vi "Autonomous Independent.vi"() -> ()   [LabVIEW 2012]
doc: "This VI is called when autonomous begins, and will automatically be terminated when autonomous ends. You can carry out timed or sensor driven robot movement independently without needing to return to the caller."
uses:
  <vilib>/Rock Robotics/WPI/SafetyOutput/WPI_SafetyOutputConfigMenu.ctl
  <vilib>/Rock Robotics/WPI/Relay/WPI_RelayValue.ctl
  Extras/Global Data.vi
  <vilib>/Rock Robotics/WPI/RobotDrive/WPI_RobotDriveGetSetRefNum.vi
panel:
  out "1M in Distance":dbl
  out "Left Encdoer":string
  out "Right Encdoer":string
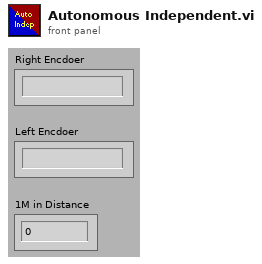
[diagram p1: front panel]
types:
  T1 = typedef "WPI_SafetyOutputConfigMenu.ctl" = enum16{"Enable", "Disable"}
  T2 = typedef "WPI_RelayDevRef.ctl" = cluster{"DevStatus":errorcluster, "Relay Channel":T3, "Digital Module":T4, "Relay Direction":T5}
  T3 = typedef "FPGA_DIORelayChannel.ctl" = enum8{"Relay 1", "Relay 2", "Relay 3", "Relay 4", "Relay 5", "Relay 6", "Relay 7", "Relay 8", "Invalid"}
  T4 = typedef "FPGA_TypedefDigitalModule.ctl" = enum16{"Digital Module 1", "Digital Module 2"}
  T5 = typedef "WPI_RelayDirection.ctl" = enum16{"Both directions", "Forward only", "Reverse only"}
  T6 = typedef "WPI_RobotDriveDevRef.ctl" = cluster{"DevStatus":errorcluster, "Motors[]":T7[], "Square Inputs":bool, "Max Output":dbl, "Isochronous":bool}
  T7 = typedef "WPI_MotorControlDeviceRef.ctl" = cluster{"DeviceStatus":errorcluster, "Type":enum16{"PWM", "CAN"}, "PWM":cluster{"Digital Module":T4, "PWM Channel":T8, "DeadBand":T9}, "CAN":cluster{"Device Number":u8, "Control Mode":T10, "Semaphore":T11, "Max Vout":dbl}, "Invert":bool, "TransformRef":T12, "InvTransformRef":T12}
  T8 = typedef "FPGA_DIOPWMChannel.ctl" = enum8{"PWM 1", "PWM 2", "PWM 3", "PWM 4", "PWM 5", "PWM 6", "PWM 7", "PWM 8", "PWM 9", "PWM 10", "Invalid"}
  T9 = typedef "WPI_PWMDeadband.ctl" = cluster{"Name":string, "maxPositivePwm":i32, "minPositivePwm":i32, "centerPwm":i32, "maxNegativePwm":i32, "minNegativePwm":i32, "angularRange":u16}
  T10 = typedef "WPI_CANJaguar_ControlMode.ctl" = enum8{"Percent VBus", "Current", "Speed", "Position", "Voltage"}
  T11 = typedef "Semaphore RefNum" = refnum<k1>
  T12 = typedef "WPI_PWMTransform_ConPane.ctl" = refnum<vi>
  T13 = typedef "WPI_DigitalInputDevRef.ctl" = cluster{"DevStatus":errorcluster, "DIO Channel":T14, "Digital Module":T4}
  T14 = typedef "FPGA_DIOChannel.ctl" = enum8{"DIO 1", "DIO 2", "DIO 3", "DIO 4", "DIO 5", "DIO 6", "DIO 7", "DIO 8", "DIO 9", "DIO 10", "DIO 11", "DIO 12", "DIO 13", "DIO 14", "Invalid"}
  T15 = typedef "WPI_RelayValue.ctl" = enum16{"Off", "On", "Forward", "Reverse"}
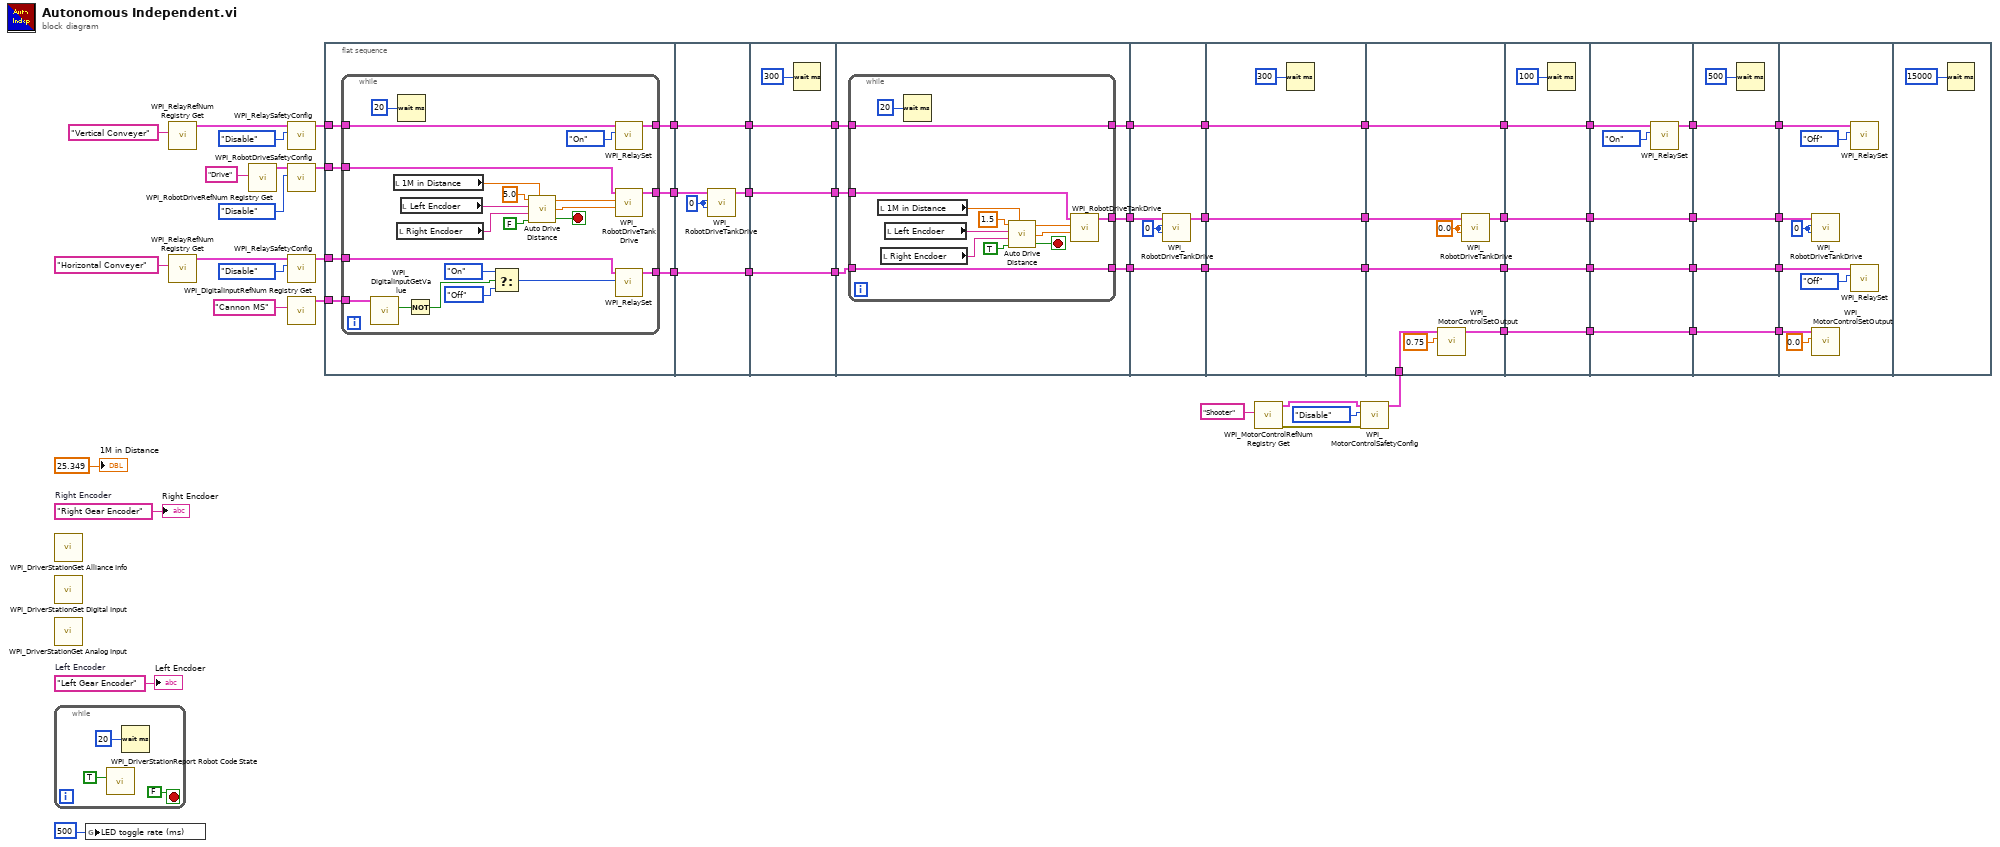
[diagram p0: block diagram]
diagram:
  w44 = "Left Gear Encoder"  # Left Encoder
  w45 = "Right Gear Encoder"  # Right Encoder
  n1 = call <vilib>:"WPI_DriverStationGet Alliance Info.vi"() -> ()  [unwired: 12 out]
  n2 = call <vilib>:"WPI_DriverStationGet Digital Input.vi"() -> ()  [unwired: 12 out]
  n3 = call <vilib>:"WPI_DriverStationGet Analog Input.vi"() -> ()  [unwired: 12 out]
  n4 = while {
    stop <- FALSE stop-if-true
    n5 = call <vilib>:"WPI_DriverStationReport Robot Code State.vi"("Autonomous"=TRUE) -> ()  [unwired: 10 in, 1 out]
    n6 = Wait (ms)(milliseconds to wait=u32 20) -> ()  [unwired: 1 out]
  }
  n7 = global write "Global Data.vi" "LED toggle rate (ms)"(u32 500 ("LED ms toggle rate")) -> ()
  n8 = call <vilib>:"WPI_RelayRefNum Registry Get.vi"("refnum name"="Vertical Conveyer") -> ("RelayDevRef"=w39:T2)  [unwired: 9 in, 1 out]
  n9 = call <vilib>:"WPI_RelayRefNum Registry Get.vi"("refnum name"="Horizontal Conveyer") -> ("RelayDevRef"=w42:T2)  [unwired: 9 in, 1 out]
  n10 = call <vilib>:"WPI_RobotDriveRefNum Registry Get.vi"("refnum name"="Drive") -> ("RobotDriveDevRef"=w54:T6)  [unwired: 9 in, 1 out]
  n11 = call <vilib>:"WPI_RelaySafetyConfig.vi"("mode"=WPI_SafetyOutputConfigMenu."Disable", "RelayDevRef"=w39) -> ("RelayDevRef"=w38:T2)  [unwired: 8 in, 1 out]
  n12 = call <vilib>:"WPI_RobotDriveSafetyConfig.vi"("mode"=WPI_SafetyOutputConfigMenu."Disable", "RobotDriveDevRef"=w54) -> ("RobotDriveDevRef"=w53:T6)  [unwired: 8 in, 1 out]
  n13 = call <vilib>:"WPI_RelaySafetyConfig.vi"("mode"=WPI_SafetyOutputConfigMenu."Disable", "RelayDevRef"=w42) -> ("RelayDevRef"=w37:T2)  [unwired: 8 in, 1 out]
  n14 = call <vilib>:"WPI_DigitalInputRefNum Registry Get.vi"("refnum name"="Cannon MS") -> ("DigitalInputDevRef"=w36:T13)  [unwired: 9 in, 1 out]
  n15 = flat-sequence {
    tunnel: w53 -> [w67]
    tunnel: w38 -> [w66]
    tunnel: w37 -> [w65]
    tunnel: w36 -> [w64]
    tunnel: [w63] -> w31
    tunnel: [w62] -> w30
    tunnel: [w61] -> w29
    tunnel: w31 -> [w93]
    tunnel: [w92] -> w51
    tunnel: w30 -> [w91]
    tunnel: w29 -> [w90]
    tunnel: [w91] -> w27
    tunnel: [w90] -> w25
    tunnel: w51 -> [w98]
    tunnel: [w98] -> w50
    tunnel: [w96] -> w28
    tunnel: w27 -> [w96]
    tunnel: [w95] -> w26
    tunnel: w25 -> [w95]
    tunnel: w50 -> [w103]
    tunnel: w28 -> [w104]
    tunnel: w26 -> [w102]
    tunnel: [w101] -> w24
    tunnel: [w100] -> w23
    tunnel: [w99] -> w22
    tunnel: [w122] -> w52
    tunnel: w24 -> [w118]
    tunnel: w23 -> [w119]
    tunnel: w22 -> [w120]
    tunnel: [w119] -> w21
    tunnel: [w118] -> w20
    tunnel: w52 -> [w123]
    tunnel: [w125] -> w3
    tunnel: w21 -> [w125]
    tunnel: [w124] -> w2
    tunnel: w20 -> [w124]
    tunnel: [w123] -> w1
    tunnel: [w134] -> w49
    tunnel: w16 -> [w132]
    tunnel: [w130] -> w15
    tunnel: [w129] -> w13
    tunnel: w3 -> [w129]
    tunnel: [w128] -> w11
    tunnel: w2 -> [w128]
    tunnel: w1 -> [w127]
    tunnel: w49 -> [w138]
    tunnel: [w138] -> w47
    tunnel: w15 -> [w135]
    tunnel: [w137] -> w14
    tunnel: w13 -> [w137]
    tunnel: [w136] -> w12
    tunnel: w11 -> [w136]
    tunnel: [w135] -> w4
    tunnel: w47 -> [w145]
    tunnel: [w145] -> w46
    tunnel: w14 -> [w143]
    tunnel: w12 -> [w141]
    tunnel: [w142] -> w9
    tunnel: [w141] -> w7
    tunnel: [w140] -> w5
    tunnel: w4 -> [w140]
    tunnel: w46 -> [w150]
    tunnel: [w150] -> w48
    tunnel: [w148] -> w10
    tunnel: w9 -> [w148]
    tunnel: [w147] -> w8
    tunnel: w7 -> [w147]
    tunnel: [w146] -> w6
    tunnel: w5 -> [w146]
    tunnel: w48 -> [w157]
    tunnel: w10 -> [w155]
    tunnel: w8 -> [w154]
    tunnel: w6 -> [w151]
    frame #0 {
      n16 = while {
        tunnel: [w89] -> w63
        tunnel: w67 -> [w84]
        tunnel: w66 -> [w79]
        tunnel: w65 -> [w78]
        tunnel: w64 -> [w76]
        tunnel: [w70] -> w62
        tunnel: [w69] -> w61
        stop <- w83 stop-if-true
        n17 = call <vilib>:"WPI_DigitalInputGetValue.vi"("DigitalInputDevRef"=w76) -> ("Value"=w75:bool)  [unwired: 8 in, 2 out]
        n18 = local read "1M in Distance"() -> (w81:dbl)
        n19 = local read "Right Encdoer"() -> (w87:string)
        n20 = Wait (ms)(milliseconds to wait=u32 20) -> ()  [unwired: 1 out]
        n21 = local read "Left Encdoer"() -> (w88:string)
        n22 = Not(x=w75) -> (.not. x?=w74:bool)
        n23 = Select(t=WPI_RelayValue."On" ("RelayValue"), s=w74, f=WPI_RelayValue."Off" ("RelayValue")) -> (s? t:f=w71:T15)
        n24 = call "Auto Drive Distance.vi"("Wanted Distance"=5.0 ("Numeric Control"), "Left Gear Encoder"=w88, "Right Gear Encoder"=w87, "Reverse?"=FALSE, "1M in Distance"=w81) -> ("Left Stick Value"=w86:dbl, "Right Stick Value"=w85:dbl, "Completed?"=w83:bool)
        n25 = call <vilib>:"WPI_RelaySet.vi"("RelayValue"=WPI_RelayValue."On", "RelayDevRef"=w79) -> ("RelayDevRef"=w70:T2)  [unwired: 8 in, 1 out]
        n26 = call <vilib>:"WPI_RobotDriveTankDrive.vi"("Right axis value"=w85, "Left axis value"=w86, "RobotDriveDevRef"=w84) -> ("RobotDriveDevRef"=w89:T6)  [unwired: 6 in, 2 out]
        n27 = call <vilib>:"WPI_RelaySet.vi"("RelayValue"=w71, "RelayDevRef"=w78) -> ("RelayDevRef"=w69:T2)  [unwired: 8 in, 1 out]
      }
    }
    frame #1 {
      w94 = 0
      n28 = call <vilib>:"WPI_RobotDriveTankDrive.vi"("Right axis value"=w94, "Left axis value"=w94, "RobotDriveDevRef"=w93) -> ("RobotDriveDevRef"=w92:T6)  [unwired: 6 in, 2 out]
    }
    frame #2 {
      n29 = Wait (ms)(milliseconds to wait=u32 300) -> ()  [unwired: 1 out]
    }
    frame #3 {
      n30 = while {
        tunnel: [w117] -> w99
        tunnel: w103 -> [w112]
        tunnel: w104 -> [w105]
        tunnel: w102 -> [w106]
        tunnel: [w106] -> w101
        tunnel: [w105] -> w100
        stop <- w111 stop-if-true
        n31 = local read "1M in Distance"() -> (w109:dbl)
        n32 = local read "Right Encdoer"() -> (w115:string)
        n33 = local read "Left Encdoer"() -> (w116:string)
        n34 = Wait (ms)(milliseconds to wait=u32 20) -> ()  [unwired: 1 out]
        n35 = call "Auto Drive Distance.vi"("Wanted Distance"=1.5 ("Numeric Control"), "Left Gear Encoder"=w116, "Right Gear Encoder"=w115, "Reverse?"=TRUE, "1M in Distance"=w109) -> ("Left Stick Value"=w114:dbl, "Right Stick Value"=w113:dbl, "Completed?"=w111:bool)
        n36 = call <vilib>:"WPI_RobotDriveTankDrive.vi"("Right axis value"=w113, "Left axis value"=w114, "RobotDriveDevRef"=w112) -> ("RobotDriveDevRef"=w117:T6)  [unwired: 6 in, 2 out]
      }
    }
    frame #4 {
      w121 = 0
      n37 = call <vilib>:"WPI_RobotDriveTankDrive.vi"("Right axis value"=w121, "Left axis value"=w121, "RobotDriveDevRef"=w120) -> ("RobotDriveDevRef"=w122:T6)  [unwired: 6 in, 2 out]
    }
    frame #5 {
      n38 = Wait (ms)(milliseconds to wait=u32 300) -> ()  [unwired: 1 out]
    }
    frame #6 {
      w133 = 0.0 ("Right axis value")
      n39 = call <vilib>:"WPI_MotorControlSetOutput.vi"("Output"=0.75, "MotorControlDevRef"=w132) -> ("MotorControlDevRef"=w130:T7)  [unwired: 7 in, 2 out]
      n40 = call <vilib>:"WPI_RobotDriveTankDrive.vi"("Right axis value"=w133, "Left axis value"=w133, "RobotDriveDevRef"=w127) -> ("RobotDriveDevRef"=w134:T6)  [unwired: 6 in, 2 out]
    }
    frame #7 {
      n41 = Wait (ms)(milliseconds to wait=u32 100) -> ()  [unwired: 1 out]
    }
    frame #8 {
      n42 = call <vilib>:"WPI_RelaySet.vi"("RelayValue"=WPI_RelayValue."On", "RelayDevRef"=w143) -> ("RelayDevRef"=w142:T2)  [unwired: 8 in, 1 out]
    }
    frame #9 {
      n43 = Wait (ms)(milliseconds to wait=u32 500) -> ()  [unwired: 1 out]
    }
    frame #10 {
      w158 = 0
      n44 = call <vilib>:"WPI_RobotDriveTankDrive.vi"("Right axis value"=w158, "Left axis value"=w158, "RobotDriveDevRef"=w157) -> ()  [unwired: 6 in, 3 out]
      n45 = call <vilib>:"WPI_MotorControlSetOutput.vi"("Output"=0.0, "MotorControlDevRef"=w151) -> ()  [unwired: 7 in, 3 out]
      n46 = call <vilib>:"WPI_RelaySet.vi"("RelayValue"=WPI_RelayValue."Off", "RelayDevRef"=w155) -> ()  [unwired: 8 in, 2 out]
      n47 = call <vilib>:"WPI_RelaySet.vi"("RelayValue"=WPI_RelayValue."Off", "RelayDevRef"=w154) -> ()  [unwired: 8 in, 2 out]
    }
    frame #11 {
      n48 = Wait (ms)(milliseconds to wait=u32 15000) -> ()  [unwired: 1 out]
    }
  }
  n49 = call <vilib>:"WPI_MotorControlRefNum Registry Get.vi"("refnum name"="Shooter") -> ("error out"=w18:errorcluster, "MotorControlDevRef"=w19:T7)  [unwired: 9 in]
  n50 = call <vilib>:"WPI_MotorControlSafetyConfig.vi"("error in (no error)"=w18, "mode"=WPI_SafetyOutputConfigMenu."Disable", "MotorControlDevRef"=w19) -> ("MotorControlDevRef"=w16:T7)  [unwired: 7 in, 1 out]
  "Right Encdoer" <- w45
  "Left Encdoer" <- w44
  "1M in Distance" <- 25.349
